vi "字符串操作函数（二）.vi"() -> ()   [LabVIEW 2010]
panel:
  out "被替换部分":string
  out "替换结果":string
  out "被替换部分":string
  out "替换结果":string
  out "替换结果":string
  out "被替换部分":string
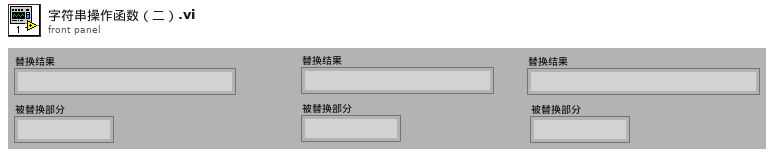
[diagram p1: front panel]
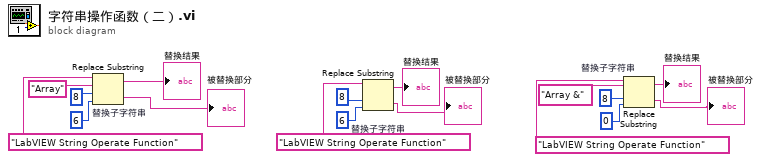
[diagram p0: block diagram]
diagram:
  n1 = Replace Substring "替换子字符串"(2:6, 3:8, 4:"Array", 5:"LabVIEW String Operate Function") -> (0:→"被替换部分":string, 1:→"替换结果":string)
  n2 = Replace Substring "替换子字符串"(2:6, 3:8, 5:"LabVIEW String Operate Function") -> (0:→"被替换部分":string, 1:→"替换结果":string)  [unwired: 1 in]
  n3 = Replace Substring "替换子字符串"(2:0, 3:8, 4:"Array &", 5:"LabVIEW String Operate Function") -> (0:→"被替换部分":string, 1:→"替换结果":string)
